vi "PPG_ABC.pattern data 2 byte array.vi"(1 "PGData":T2) -> (15 "byteArray out":T1)   [LabVIEW 2014, in "PPG_ABC.lvlib"]
doc: "Converts data from \"PGDataType\" to a byte array. This method is specific for using user defined patterns constructed of characters as used by the MM6 class."
uses:
  PPG_ABC.lvlib
  PPG_ABC.PG_dataType.ctl
  CS_Core/CSSystem/CoreDefs/CoreDefs.rawDataType.ctl
  CS_Core/CSSystem/CoreLib/CoreLib.string 2 byte array.vi
  CS_Core/CSSystem/CoreLib/CoreLib.int 2 byte array.vi
  CS_Core/CSSystem/CoreLib/CoreLib.double array 2 byte array.vi
  CS_Core/CSSystem/CoreLib/CoreLib.lvlib
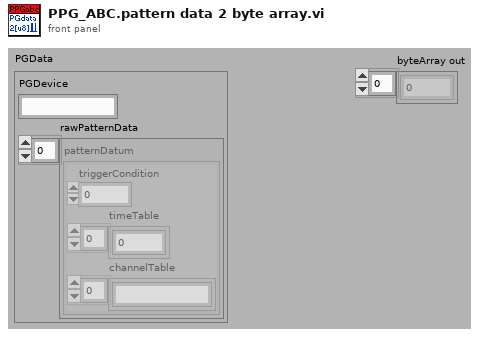
[diagram p1: front panel]
types:
  T1 = typedef "CoreDefs.rawDataType.ctl" = i8[]
  T2 = typedef "PPG_ABC.lvlib/PPG_ABC.PG_dataType.ctl" = cluster{"PGDevice":string, "rawPatternData":cluster{"triggerCondition":i32, "timeTable":dbl[], "channelTable":string[]}[]}
  T3 = cluster{"triggerCondition":i32, "timeTable":dbl[], "channelTable":string[]}[]
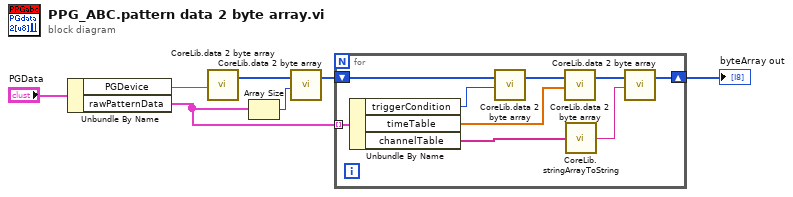
[diagram p0: block diagram]
diagram:
  n1 = Unbundle By Name("PGData") -> ("PGDevice"=w6:string, "rawPatternData"=w2:T3)
  n2 = call-poly "CoreLib.data 2 byte array.vi"("string"=w6) -> ("byteArray out"=w4:T1)  [unwired: 18 in]
  n3 = Array Size(array=w2) -> (size(s)=w1:i32)
  n4 = call-poly "CoreLib.data 2 byte array.vi"("byteArray"=w4, "i32"=w1) -> ("byteArray out"=w3:T1)  [unwired: 17 in]
  n5 = for {
    tunnel: w2 -> [w16] mode=indexing
    shift-right: [w8] -> w5
    shift-left: w3 -> [w11]
    n6 = Unbundle By Name(w16) -> ("triggerCondition"=w15:i32, "timeTable"=w14:dbl[], "channelTable"=w13:string[])
    n7 = call-poly "CoreLib.data 2 byte array.vi"("byteArray"=w11, "i32"=w15) -> ("byteArray out"=w10:T1)  [unwired: 17 in]
    n8 = call-poly "CoreLib.data 2 byte array.vi"("byteArray"=w10, "[d64]"=w14) -> ("byteArray out"=w9:T1)  [unwired: 17 in]
    n9 = call "CoreLib.stringArrayToString.vi"("Array"=w13) -> ("String"=w12:string)
    n10 = call-poly "CoreLib.data 2 byte array.vi"("byteArray"=w9, "string"=w12) -> ("byteArray out"=w8:T1)  [unwired: 17 in]
  }
  "byteArray out" <- w5
